vi "CTD.vi"(0 "CTD":bool, 2 "PV":i32, 3 "Reset":bool) -> (14 "Q":bool, 15 "CT":i32)   [LabVIEW 2020]
uses:
  7b58aaaf-3230-4726-a54c-2c8544926117.vi
panel:
  out "mem ct":i32
  out "Mem":bool
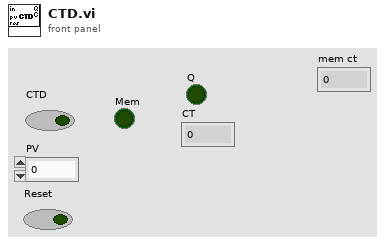
[diagram p1: front panel]
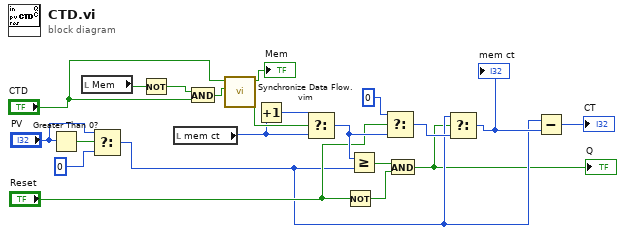
[diagram p0: block diagram]
diagram:
  n1 = Greater Than 0?(x="PV") -> (x > 0?=w21:bool)
  n2 = local read "Mem"() -> (w12:bool)
  n3 = Select(t="PV", s=w21, f=0) -> (s? t:f=w3:i32)
  n4 = Not(x=w12) -> (.not. x?=w13:bool)
  n5 = local read "mem ct"() -> (w4:i32)
  n6 = And(x=w13, y="CTD") -> (x .and. y?=w18:bool)
  n7 = call "Synchronize Data Flow.vim"("input 2"=w18, "input 1"="CTD") -> ("output 2"=w15:bool, "output 1"=→"Mem":bool)  [unwired: 2 in, 2 out]
  n8 = Increment(x=w4) -> (x+1=w14:i32)
  n9 = Select(t=w14, s=w15, f=w4) -> (s? t:f=w10:i32)
  n10 = Not(x="Reset") -> (.not. x?=w11:bool)
  n11 = Greater Or Equal?(x=w10, y=w3) -> (x >= y?=w8:bool)
  n12 = Select(t=0, s="Reset", f=w10) -> (s? t:f=w7:i32)
  n13 = And(x=w8, y=w11) -> (x .and. y?=w1:bool)
  "Q" <- w1
  n14 = Select(t=w3, s=w1, f=w7) -> (s? t:f=w5:i32)
  "mem ct" <- w5
  n15 = Subtract(x=w3, y=w5) -> (x-y=→"CT":i32)
